vi "noslimites.vi"(8 "lim":dbl, 10 "PVx":dbl, 11 "SPx:":dbl) -> (3 "Está dentro dos limites?":bool)   [LabVIEW 2019]
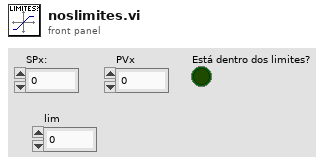
[diagram p1: front panel]
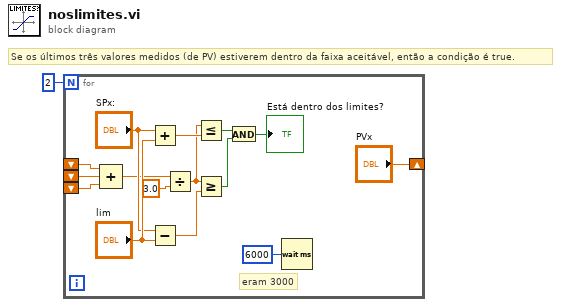
[diagram p0: block diagram]
diagram:
  # "Se os últimos três valores medidos (de PV) estiverem dentro da faixa aceitável, então a condição é true."
  n1 = for {
    N: 2 -> [_]
    shift-right: ["PVx"] -> _
    shift-left: _ -> [w9]
    shift-left: _ -> [w8]
    shift-left: _ -> [w7]
    # "eram 3000"
    n2 = Compound Arithmetic op=ADD(w9, w8, w7) -> (w6:dbl)
    n3 = Add(x="SPx:", y="lim") -> (x+y=w15:dbl)
    n4 = Subtract(x="SPx:", y="lim") -> (x-y=w16:dbl)
    n5 = Divide(x=w6, y=3.0) -> (x/y=w3:dbl)
    n6 = Less Or Equal?(x=w3, y=w15) -> (x <= y?=w13:bool)
    n7 = Greater Or Equal?(x=w3, y=w16) -> (x >= y?=w14:bool)
    n8 = And(x=w13, y=w14) -> (x .and. y?=→"Está dentro dos limites?":bool)
    n9 = Wait (ms)(milliseconds to wait=u32 6000) -> ()  [unwired: 1 out]
  }
